vi "Decode_RAW_to_DEC_171213.vi"(1 "read buffer":string) -> (0 "DEC SGL output":sgl[][](array[numeric]))   [LabVIEW 2016]
panel:
  out "transposed array":sgl[][](array[numeric])
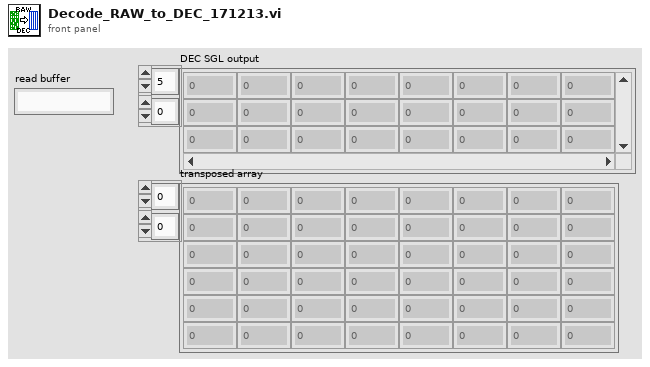
[diagram p1: front panel]
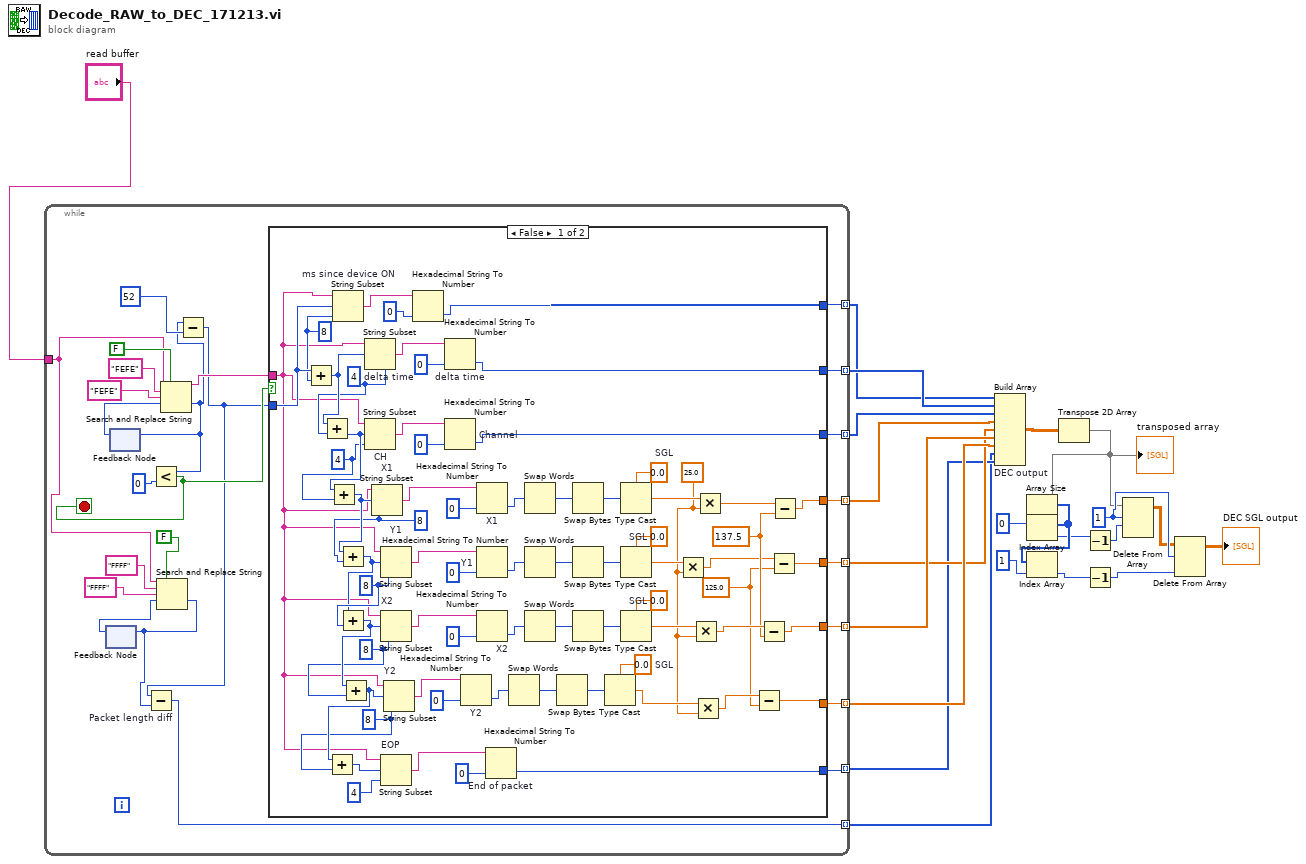
[diagram p0: block diagram]
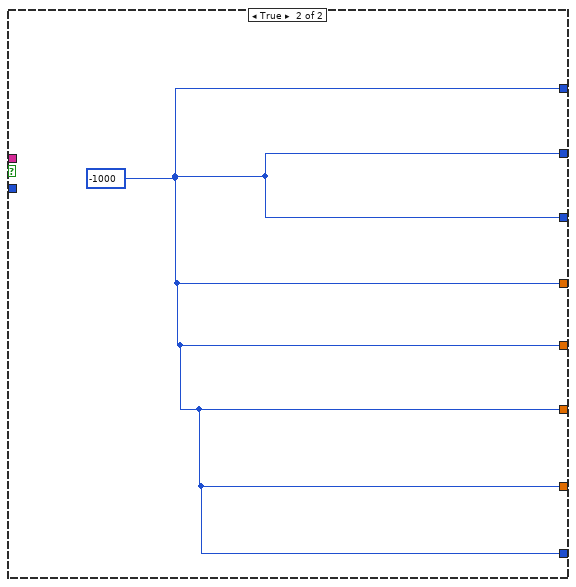
[diagram p2: hidden frame]
diagram:
  w18 = 1 ("length")
  n1 = while {
    tunnel: "read buffer" -> [w29]
    tunnel: [w41] -> w5 mode=indexing
    tunnel: [w39] -> w6 mode=indexing
    tunnel: [w38] -> w7 mode=indexing
    tunnel: [w37] -> w8 mode=indexing
    tunnel: [w36] -> w9 mode=indexing
    tunnel: [w35] -> w10 mode=indexing
    tunnel: [w34] -> w11 mode=indexing
    tunnel: [w33] -> w2 mode=indexing
    tunnel: [w26] -> w1 mode=indexing
    stop <- w40 stop-if-true
    n2 = feedback #1() -> (w28:i32)  [unwired: 1 in]
    n3 = feedback #2() -> (w44:i32)  [unwired: 1 in]
    n4 = Search and Replace String(replace all?=FALSE ("replace all? (F)"), input string=w29, search string="FFFF", replace string="FFFF" ("replace string (\"\")"), offset=w28) -> (offset past replacement=w25:i32)  [unwired: 3 in, 3 out]
    n5 = feedback-in #1(w25) -> ()
    n6 = Search and Replace String(replace all?=FALSE ("replace all? (F)"), input string=w29, search string="FEFE", replace string="FEFE" ("replace string (\"\")"), offset=w44) -> (result string=w42:string, offset past replacement=w24:i32)  [unwired: 3 in, 2 out]
    n7 = feedback-in #2(w24) -> ()
    n8 = Less?(x=w24, y=0) -> (x < y?=w40:bool)
    n9 = Subtract(x=w24, y=52) -> (x-y=w23:i32)
    n10 = Subtract "Packet length diff"(x=w23, y=w25) -> (x-y=w26:i32)
    n11 = case shown="False" w40 {
      tunnel: w42 -> [w99 _]
      tunnel: [w96 w116] -> w41
      tunnel: w23 -> [w115 _]
      tunnel: [w93 w116] -> w39
      tunnel: [w90 w116] -> w38
      tunnel: [w57 w116] -> w37
      tunnel: [w52 w116] -> w36
      tunnel: [w55 w116] -> w35
      tunnel: [w50 w116] -> w34
      tunnel: [w59 w116] -> w33
      frame False {
        w48 = sgl 125.0 ("Half-height of the sensor board")
        w53 = sgl 137.5 ("Half-width of the sensor board")
        w58 = sgl 25.0 ("y")
        w65 = sgl 0.0  # SGL
        w72 = sgl 0.0  # SGL
        w79 = sgl 0.0  # SGL
        w85 = sgl 0.0  # SGL
        w101 = 8 ("length (rest)")
        w104 = 8 ("length (rest)")
        w107 = 8 ("length (rest)")
        w108 = 8 ("length (rest)")
        w110 = 4 ("length (rest)")
        w112 = 4 ("length (rest)")
        w114 = 8 ("length (rest)")
        n12 = Add(x=w115, y=w114) -> (x+y=w113:i32)
        n13 = Add(x=w113, y=w112) -> (x+y=w111:i32)
        n14 = Add(x=w111, y=w110) -> (x+y=w109:i32)
        n15 = String Subset "ms since device ON"(string=w99, offset (0)=w115, length (rest)=w114) -> (substring=w98:string)
        n16 = Add(x=w109, y=w108) -> (x+y=w106:i32)
        n17 = Add(x=w106, y=w107) -> (x+y=w105:i32)
        n18 = Add(x=w105, y=w104) -> (x+y=w102:i32)
        n19 = Add(x=w102, y=w101) -> (x+y=w103:i32)
        n20 = String Subset "delta time"(string=w99, offset (0)=w113, length (rest)=w112) -> (substring=w94:string)
        n21 = String Subset "CH"(string=w99, offset (0)=w111, length (rest)=w110) -> (substring=w91:string)
        n22 = String Subset "X1"(string=w99, offset (0)=w109, length (rest)=w108) -> (substring=w89:string)
        n23 = String Subset "Y1"(string=w99, offset (0)=w106, length (rest)=w107) -> (substring=w77:string)
        n24 = String Subset "X2"(string=w99, offset (0)=w105, length (rest)=w104) -> (substring=w70:string)
        n25 = String Subset "EOP"(string=w99, offset (0)=w103, length (rest)=4 ("length (rest)")) -> (substring=w60:string)
        n26 = String Subset "Y2"(string=w99, offset (0)=w102, length (rest)=w101) -> (substring=w63:string)
        n27 = Hexadecimal String To Number ("ms since ON")(string=w98, default (0uL)=u32 0 ("default (0 U32)")) -> (number=w96:u32)  [unwired: 1 in, 1 out]
        n28 = Hexadecimal String To Number "delta time"(string=w94, default (0uL)=u32 0 ("default (0 U32)")) -> (number=w93:u32)  [unwired: 1 in, 1 out]
        n29 = Hexadecimal String To Number "Channel"(string=w91, default (0uL)=u32 0 ("default (0 U32)")) -> (number=w90:u32)  [unwired: 1 in, 1 out]
        n30 = Hexadecimal String To Number "Y2"(string=w63, default (0uL)=u32 0 ("default (0 U32)")) -> (number=w67:u32)  [unwired: 1 in, 1 out]
        n31 = Hexadecimal String To Number "X1"(string=w89, default (0uL)=u32 0 ("default (0 U32)")) -> (number=w87:u32)  [unwired: 1 in, 1 out]
        n32 = Hexadecimal String To Number "Y1"(string=w77, default (0uL)=u32 0 ("default (0 U32)")) -> (number=w81:u32)  [unwired: 1 in, 1 out]
        n33 = Hexadecimal String To Number "X2"(string=w70, default (0uL)=u32 0 ("default (0 U32)")) -> (number=w74:u32)  [unwired: 1 in, 1 out]
        n34 = Hexadecimal String To Number "End of packet"(string=w60, default (0uL)=u32 0 ("default (0 U32)")) -> (number=w59:u32)  [unwired: 1 in, 1 out]
        n35 = Swap Words(1:w67) -> (0:w66:u32)
        n36 = Swap Words(1:w87) -> (0:w86:u32)
        n37 = Swap Words(1:w81) -> (0:w80:u32)
        n38 = Swap Words(1:w74) -> (0:w73:u32)
        n39 = Swap Bytes(anything=w66) -> (byte swapped=w64:u32)
        n40 = Swap Bytes(anything=w86) -> (byte swapped=w84:u32)
        n41 = Swap Bytes(anything=w80) -> (byte swapped=w78:u32)
        n42 = Swap Bytes(anything=w73) -> (byte swapped=w71:u32)
        n43 = Type Cast(type=w65, x=w64) -> (*(type *) &x=w62:sgl)
        n44 = Type Cast(type=w85, x=w84) -> (*(type *) &x=w83:sgl)
        n45 = Type Cast(type=w79, x=w78) -> (*(type *) &x=w76:sgl)
        n46 = Type Cast(type=w72, x=w71) -> (*(type *) &x=w69:sgl)
        n47 = Multiply(x=w76, y=w58) -> (x*y=w51:sgl)
        n48 = Multiply(x=w69, y=w58) -> (x*y=w54:sgl)
        n49 = Multiply(x=w62, y=w58) -> (x*y=w49:sgl)
        n50 = Multiply(x=w83, y=w58) -> (x*y=w56:sgl)
        n51 = Subtract(x=w49, y=w48) -> (x-y=w50:sgl)
        n52 = Subtract(x=w54, y=w53) -> (x-y=w55:sgl)
        n53 = Subtract(x=w51, y=w48) -> (x-y=w52:sgl)
        n54 = Subtract(x=w56, y=w53) -> (x-y=w57:sgl)
      }
      frame True {
        w116 = -1000
      }
    }
  }
  n55 = Build Array "DEC output"(w5, w6, w7, w8, w9, w10, w11, w1, w2) -> (w12:sgl[][])
  n56 = Transpose 2D Array(2D array=w12) -> (transposed array=w13:sgl[][])
  "transposed array" <- w13
  n57 = Array Size(array=w13) -> (size(s)=w20:i32[])
  n58 = Index Array(array=w20, index=0) -> (element=w15:i32)
  n59 = Index Array(array=w20, index=1) -> (element=w21:i32)
  n60 = Decrement(x=w15) -> (x-1=w16:i32)
  n61 = Decrement(x=w21) -> (x-1=w22:i32)
  n62 = Delete From Array(array=w13, length=w18, index (row)=w16) -> (array with subset deleted=w17:sgl[][])  [unwired: 1 in, 1 out]
  n63 = Delete From Array(array=w17, length=w18, index (col)=w22) -> (array with subset deleted=→"DEC SGL output":sgl[][])  [unwired: 1 in, 1 out]
